vi "EJEM8.vi"() -> ()   [LabVIEW 2013]
panel:
  out "XY Graph":cluster{dbl[], dbl[]}(graph)
  in  "Numeric":i32
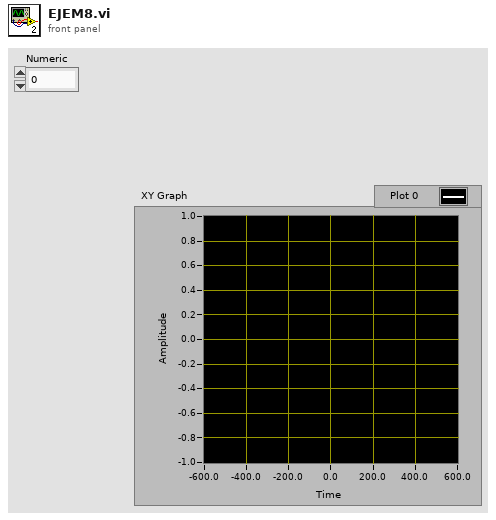
[diagram p1: front panel]
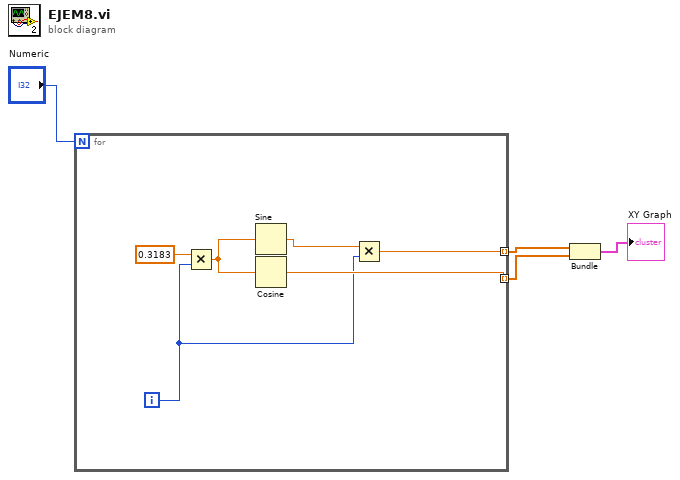
[diagram p0: block diagram]
diagram:
  n1 = for {
    N: "Numeric" -> [_]
    tunnel: [w7] -> w3 mode=indexing
    tunnel: [w6] -> w2 mode=indexing
    i -> [w5]
    n2 = Multiply(x=0.3183, y=w5) -> (x*y=w9:dbl)
    n3 = Sine(x=w9) -> (sin(x)=w8:dbl)
    n4 = Cosine(x=w9) -> (cos(x)=w7:dbl)
    n5 = Multiply(x=w8, y=w5) -> (x*y=w6:dbl)
  }
  n6 = Bundle(w2, w3) -> (→"XY Graph":cluster{dbl[], dbl[]})  [unwired: 1 in]
